vi "initialise.vi"(8 "error in (no error)":errorcluster, 11 "FPGA_AK101022Resonance in":refnum<class "FPGAWrapperAK101022Resonance.lvclass">) -> (0 "error out":errorcluster, 3 "FPGA_AK101022Resonance out":refnum<class "FPGAWrapperAK101022Resonance.lvclass">)   [LabVIEW 2010, in "FPGAWrapperAK101022Resonance.lvclass"]
uses:
  FPGAWrapperAK101022Resonance.lvclass
  GenericFPGAWrapper/GenericFPGAWrapper/GenericFPGAWrapper.lvclass
  scan_specification_cluster.ctl
  grabber/config_data_cluster.ctl
  FPGAWrapperAK101022Resonance.lvclass/FPGAWrapperAK101022Resonance.ctl
  class_data.vi
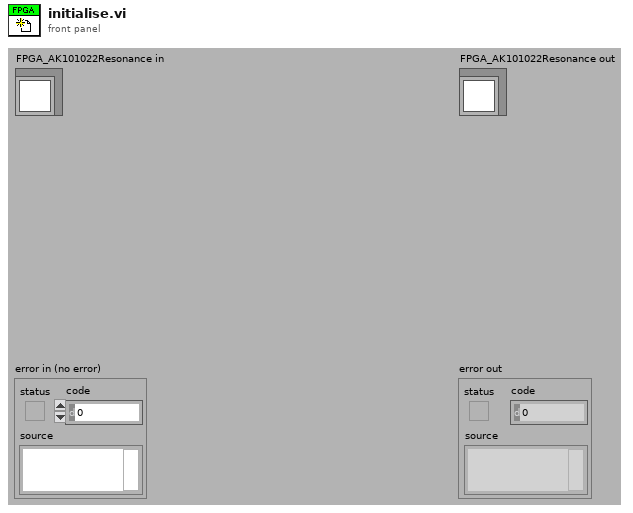
[diagram p1: front panel]
types:
  T1 = typedef "scan_specification_cluster.ctl" = cluster{"x amplitude":u16, "x resolution (pixels)":u16, "x offset fly-forward (iterations)":u16, "x offset fly-back (iterations)":u16, "y resolution (nr. of lines)":u16, "y step size":u16, "iterations per pixel":u16, "number of frames":i32, "y offset (pixels)":u16, "number of y-brake lines  (before y-fly-back)":u16, "number y-brake lines (after y-fly-back)":u16, "number of y-fly-back steps":u16, "lines per z step":u16, "number of z/intensity tuples":u16, "number of repetitions (volumes or planes)":i32, "z step size derived":u16, "choose the beginning of z scan":bool, "number of frames (settings)":i32, "FPGA trajectory?":bool}
  T2 = typedef "config_data_cluster.ctl" = cluster{"channel offsets":u32[], "invert channel?":bool[], "ADC clock phase":i32, "z/intensity memory size":i32}
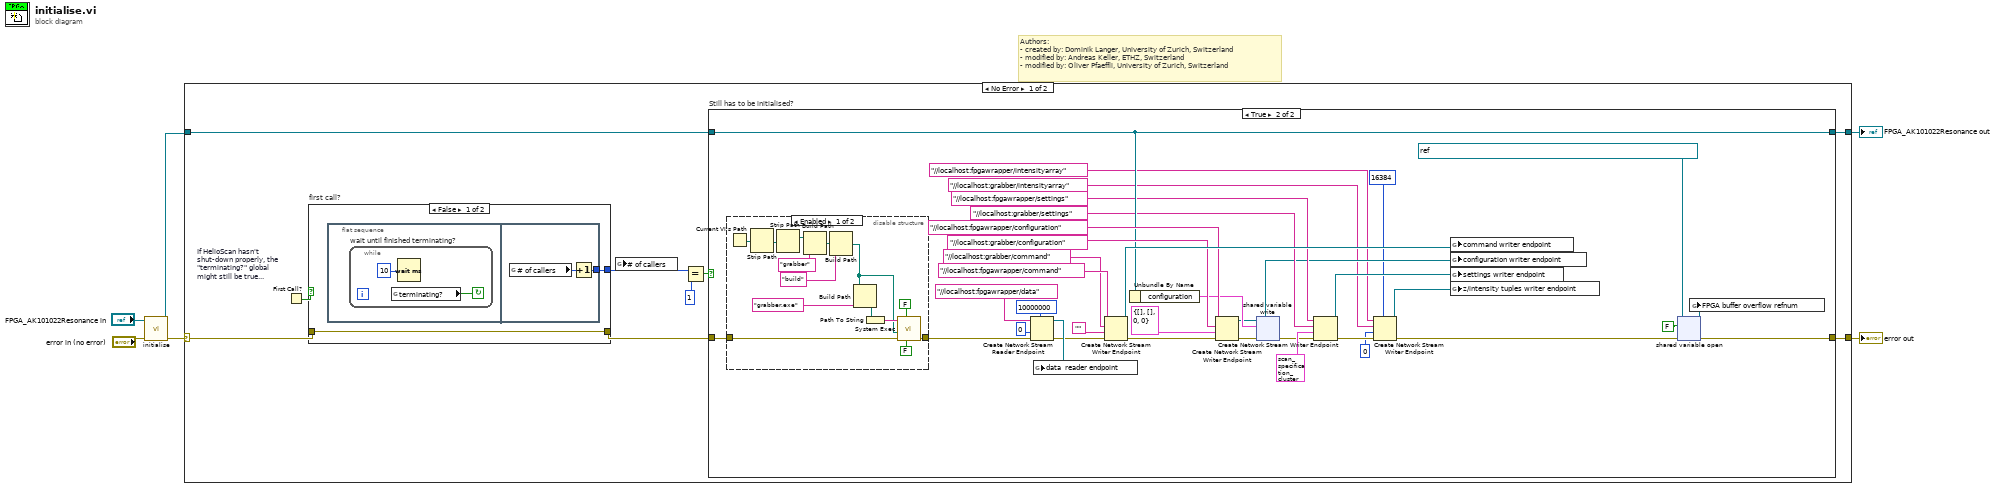
[diagram p0: block diagram]
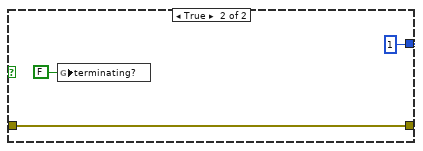
[diagram p2: hidden frame]
diagram:
  # "Authors: \n- created by: Dominik Langer, University of Zurich, Switzerland\n- modified by: Andreas Keller, ETHZ, Switzerland\n- modified by: Oliver Pfaeffli, University of Zurich, Switzerland"
  n1 = call-parent "initialise.vi"("error in (no error)"="error in (no error)", "GenericPlugin in"="FPGA_AK101022Resonance in") -> ("error out"=w2:errorcluster, "GenericPlugin out"=w1:refnum<class "FPGAWrapperAK101022Resonance.lvclass">)  [unwired: 8 in]
  n2 = case shown="No Error" w2 {
    selector: w2 -> [w8 w79]
    tunnel: [w15 w79] -> w6
    tunnel: w1 -> [w7 w78]
    tunnel: [w9 w78] -> w5
    frame No Error {
      n3 = First Call? "If HelioScan hasn't shut-down properly, the \"terminating?\" global might still be true..."() -> (First Call?: T/F=w14:bool)
      n4 = case "first call?" shown="False" w14 {
        tunnel: [w17 1 ("# of callers")] -> w12
        tunnel: [w16 w23] -> w13
        tunnel: w8 -> [w16 w23]
        frame False {
          n5 = flat-sequence {
            tunnel: [w21] -> w17
            frame #0 {
              n6 = while "wait until finished terminating?" {
                stop <- w18 continue-if-true
                n7 = global read "class_data.vi" "terminating?"() -> (w18:bool)
                n8 = Wait (ms)(milliseconds to wait=u32 10) -> ()  [unwired: 1 out]
              }
            }
            frame #1 {
              n9 = global read "class_data.vi" "# of callers"() -> (w20:i32)
              n10 = Increment(x=w20) -> (x+1=w21:i32)
            }
          }
        }
        frame True {
          n11 = global write "class_data.vi" "terminating?"(FALSE ("terminating?")) -> ()
        }
      }
      n12 = global write "class_data.vi" "# of callers"(w12) -> ()
      n13 = Equal?(x=w12, y=1) -> (x = y?=w10:bool)
      n14 = case "Still has to be initialised?" shown="True" w10 {
        tunnel: w13 -> [w26 w62]
        tunnel: [w26 w46] -> w15
        tunnel: w7 -> [w25 w43]
        tunnel: [w25 w43] -> w9
        frame False {
        }
        frame True {
          n15 = disable-structure shown="Enabled" {
            disable-tunnel: w62 -> [w70 w77]
            disable-tunnel: [w69 w77] -> w54
            frame Enabled {
              n16 = Current VI's Path() -> (path=w68:path)
              n17 = Strip Path(path=w68) -> (stripped path=w67:path)  [unwired: 1 out]
              n18 = Strip Path(path=w67) -> (stripped path=w66:path)  [unwired: 1 out]
              n19 = Build Path(base path=w66, name or relative path="grabber") -> (appended path=w65:path)
              n20 = Build Path(base path=w65, name or relative path="build") -> (appended path=w63:path)
              n21 = Build Path(base path=w63, name or relative path="grabber.exe" ("command line")) -> (appended path=w74:path)
              n22 = Path To String(path=w74) -> (string=w73:string)
              n23 = call <vilib>:"System Exec.vi"("run minimized? (F)"=FALSE, "wait until completion? (T)"=FALSE, "error in (no error)"=w70, "working directory"=w63, "command line"=w73) -> ("error out"=w69:errorcluster)  [unwired: 3 in, 3 out]
            }
            frame Disabled {
            }
          }
          n24 = Create Network Stream Reader Endpoint(7:10000000 ("reader buffer size"), 8:w54, 9:u32 0, 11:"//localhost:fpgawrapper/data" ("writer name")) -> (0:w51:errorcluster, 3:w59:refnum<k21>)  [unwired: 2 in]
          n25 = global write "class_data.vi" "data  reader endpoint"(w59) -> ()
          n26 = Create Network Stream Writer Endpoint(8:w51, 9:"", 10:"//localhost:grabber/command" ("reader url"), 11:"//localhost:fpgawrapper/command" ("writer name")) -> (0:w48:errorcluster, 3:w50:refnum<k21>)  [unwired: 2 in]
          n27 = Unbundle By Name(w43) -> ("configuration"=w42:T2)
          n28 = Create Network Stream Writer Endpoint(8:w48, 9:T2 {"channel offsets"=[], "invert channel?"=[], "ADC clock phase"=0, "z/intensity memory size"=0} ("configuration"), 10:"//localhost:grabber/configuration" ("reader url"), 11:"//localhost:fpgawrapper/configuration" ("writer name")) -> (0:w37:errorcluster, 3:w35:refnum<k21>)  [unwired: 2 in]
          n29 = shared-variable-write(w35, w37, w42) -> (w39:refnum<k21>, w36:errorcluster)  [unwired: 1 in, 1 out]
          n30 = Create Network Stream Writer Endpoint(8:w36, 9:T1 {"x amplitude"=0, "x resolution (pixels)"=0, "x offset fly-forward (iterations)"=0, "x offset fly-back (iterations)"=0, "y resolution (nr. of lines)"=0, "y step size"=0, "iterations per pixel"=0, "number of frames"=0, "y offset (pixels)"=0, "number of y-brake lines  (before y-fly-back)"=0, "number y-brake lines (after y-fly-back)"=0, "number of y-fly-back steps"=0, "lines per z step"=0, "number of z/intensity tuples"=0, "number of repetitions (volumes or planes)"=0, "z step size derived"=0, "choose the beginning of z scan"=FALSE, "number of frames (settings)"=0, "FPGA trajectory?"=FALSE} ("scan specification"), 10:"//localhost:grabber/settings" ("reader url"), 11:"//localhost:fpgawrapper/settings" ("writer name")) -> (0:w33:errorcluster, 3:w34:refnum<k21>)  [unwired: 2 in]
          n31 = Create Network Stream Writer Endpoint(7:16384 ("writer buffer size"), 8:w33, 9:u32 0, 10:"//localhost:grabber/intensityarray" ("reader url"), 11:"//localhost:fpgawrapper/intensityarray" ("writer name")) -> (0:w27:errorcluster, 3:w29:refnum<k21>)  [unwired: 1 in]
          n32 = global write "class_data.vi" "command writer endpoint"(w50) -> ()
          n33 = global write "class_data.vi" "configuration writer endpoint"(w39) -> ()
          n34 = global write "class_data.vi" "settings writer endpoint"(w34) -> ()
          n35 = global write "class_data.vi" "z/intensity tuples writer endpoint"(w29) -> ()
          n36 = shared-variable-open(refnum<k21> "ni.var.psp://localhost/grabber variables/FPGA buffer overflow%3F" ("shared variable refnum in"), w27, FALSE) -> (w55:refnum<k21>, w46:errorcluster)  [unwired: 1 in]
          n37 = global write "class_data.vi" "FPGA buffer overflow refnum"(w55) -> ()
        }
      }
    }
    frame Error {
    }
  }
  "error out" <- w6
  "FPGA_AK101022Resonance out" <- w5
